vi "provide_information_text.vi"(8 "error in (no error)":errorcluster) -> (0 "error out":errorcluster, 4 "Text out":string)   [LabVIEW 2010, in "ErrorController.lvclass"]
uses:
  ErrorController.lvclass
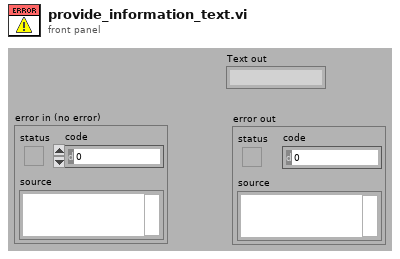
[diagram p1: front panel]
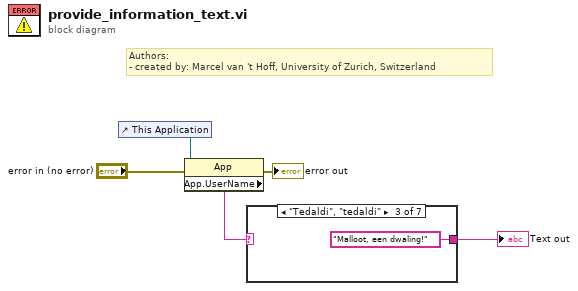
[diagram p0: block diagram]
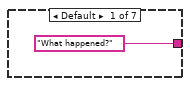
[diagram p2: hidden frame]
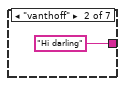
[diagram p3: hidden frame]
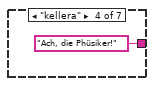
[diagram p4: hidden frame]
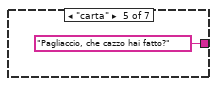
[diagram p5: hidden frame]
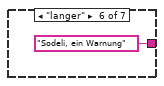
[diagram p6: hidden frame]
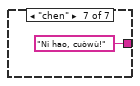
[diagram p7: hidden frame]
diagram:
  # "Authors: \n- created by: Marcel van 't Hoff, University of Zurich, Switzerland"
  n1 = control-ref of="This Application"() -> (w5:refnum<vi>)
  n2 = property class="App"(reference=w5, error in="error in (no error)") -> (error out=→"error out":errorcluster, "App.UserName"=w3:string)  [unwired: 1 out]
  n3 = case shown="\"Tedaldi\", \"tedaldi\"" w3 {
    tunnel: ["What happened?" ("App.UserName") "Hi darling" ("App.UserName") "Malloot, een dwaling!" ("App.UserName") "Ach, die Phüsiker!" ("App.UserName") "Pagliaccio, che cazzo hai fatto?" ("App.UserName") "Sodeli, ein Warnung" ("App.UserName") "Ni hao, cuòwù!" ("App.UserName")] -> w2
    frame Default {
    }
    frame "vanthoff" {
    }
    frame "Tedaldi", "tedaldi" {
    }
    frame "kellera" {
    }
    frame "carta" {
    }
    frame "langer" {
    }
    frame "chen" {
    }
  }
  "Text out" <- w2
